vi "GSI-HVSwitch2.set operational mode.vi"(0 "i ref in":refnum<vi>, 2 "mode":T1, 3 "ms timeout (10000)":i32=10000, 5 "error in (no error)":errorcluster) -> (14 "i ref out":refnum<vi>, 17 "timed out":bool, 19 "error out":errorcluster)   [LabVIEW 2014, in "GSI-HVSwitch2.lvlib"]
doc: "Sets the operational mode of the device."
uses:
  GSI-HVSwitch2.lvlib
  GSI-HVSwitch2.mode.ctl
  CS_Core/CSApplicationBaseClasses/DeviceBase/DeviceBase.deviceState.ctl
  CS_Core/CSApplicationBaseClasses/PSChannelBase/PSChannelBase.statusType.ctl
  CSlibraries/UtilityLib/UtilityLib.valueStatus.ctl
  CS_Core/CSSystem/CoreDefs/CoreDefs.error_type.ctl
  CS_Core/CSSystem/CoreDefs/CoreDefs.error_severity.ctl
  CS_Core/CSApplicationBaseClasses/DeviceBase/DeviceBase.lvlib
  CS_Core/CSApplicationBaseClasses/PSChannelBase/PSChannelBase.lvlib
  CSlibraries/UtilityLib/UtilityLib.lvlib
  CS_Core/CSSystem/CSSystemLib/CSSystemLib.lvlib
  CS_Core/CSSystem/CoreLib/CoreLib.lvlib
  CSlibraries-extern/DimLVEvent/LVDimInterface/LVDimInterface.lvlib
  instr.lib/hvSwitch2/HVSwitch2Driver.lvlib
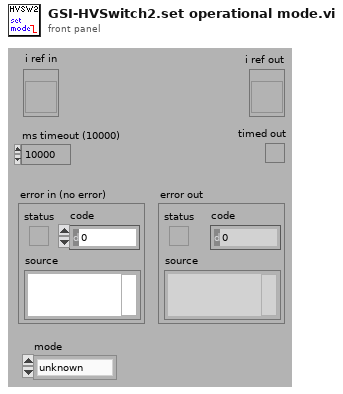
[diagram p1: front panel]
types:
  T1 = typedef "GSI-HVSwitch2.lvlib/GSI-HVSwitch2.mode.ctl" = enum16{"unknown", "switch", "stepper"}
  T2 = typedef "UtilityLib.lvlib/UtilityLib.valueStatus.ctl" = enum16{"no info available", "stand by/off", "on", "warning", "alarm/malfunction", "not implemented", "user action required", "important information", "system default", "control default", "indicator default", "button default"}
  T3 = typedef "CoreDefs.error_severity.ctl" = enum16{"undefined", "information", "warning", "error", "fatal"}
  T4 = typedef "CoreDefs.error_type.ctl" = enum16{"no error", "can't load process", "can't unload process", "process does not exist", "can't install process", "can't remove process", "unknown function", "time out", "can't execute function", "duplicate queue name", "super not found", "caller queue invalid", "can't ping process", "unknown error", "VISA Error", "VISA timeout", "GPIB timeout", "GPIB error", "communication error", "data type mismatch", "can't read data from OPC server", "can't write data to OPC server", "OET error", "function not implemented", "process already exists", "invalid Shared Variable name", "error writing Shared Variable", "error reading Shared Variable", "invalid client name", "corrupt database", "unknown class", "call not authorized", "parameter out of range", "OET timeout: can't get data to modify", "invalid queue name", "requested operation incompatible with current state", "event undefined", "event disabled", "state undefined", "caller is not a friend", "EventBuilder: bad eventID", "EventBuilder: no DAQ devices", "a thread must not stop itself", "UNUSED ELEMENT4", "DiscArchiver: eventData incomplete", "DiscArchiver: eventData does not belong to run", "DiscArchiver: can't open file", "DiscArchiver: can't write to file", "DiscArchiver: available disc space low", "can't acquire semaphore", "error reading data from database", "notifier object is not existing", "can't register process", "can't unregister process", "illegal event type", "object disabled", "object already exists", "can't change state", "Instrument not found", "no connection to remote node", "invalid reference", "N/A", "UNUSED ELEMENT 1", "element not found", "illegal TCP/IP connection detected", "object does not exist", "invalid access ID", "unknown CS system", "invalid privilige", "unsupported data type", "unsupported server type", "IO server already exists", "Shared Variable already exists"}
  T5 = typedef "GSI-HVSwitch2.lvlib/GSI-HVSwitch2.i attribute.ctl" = cluster{"SDEX VISA Cluster":T6, "SetVoltage SW0":dbl, "SetVoltage SW1":dbl, "ActTempAmp":dbl, "ActTempPS1":dbl, "ActTempPS2":dbl, "mode":T1, "interfaceInitialized":bool, "serviceIDs":cluster{"nomVoltage0ID":i32, "nomVoltage1ID":i32, "actTempAmpID":i32, "actTempPS1ID":i32, "actTempPS2ID":i32, "modeID":i32}, "usedChannels":i32}
  T6 = typedef "SDEXDriver.lvlib/SDEX.VISA Control.ctl" = cluster{"VISA resource name":refnum<visa-resource-name>, "HEX address":u16, "VISA Timeout Value (1000 ms)":u32, "Lock Timeout (1000 ms)":u32, "semaphore":T7, "Baud rate":u32, "revision":T8, "deviceInfo":string}
  T7 = typedef "Semaphore RefNum" = refnum<k1>
  T8 = typedef "SDEXDriver.lvlib/SDEX.revisionType.ctl" = enum16{"unknown", "hvamp3", "hvswi1", "htrp0", "WDG0"}
  T9 = typedef "DeviceBase.lvlib/DeviceBase.deviceState.ctl" = i16
  T10 = typedef "PSChannelBase.lvlib/PSChannelBase.statusType.ctl" = i32
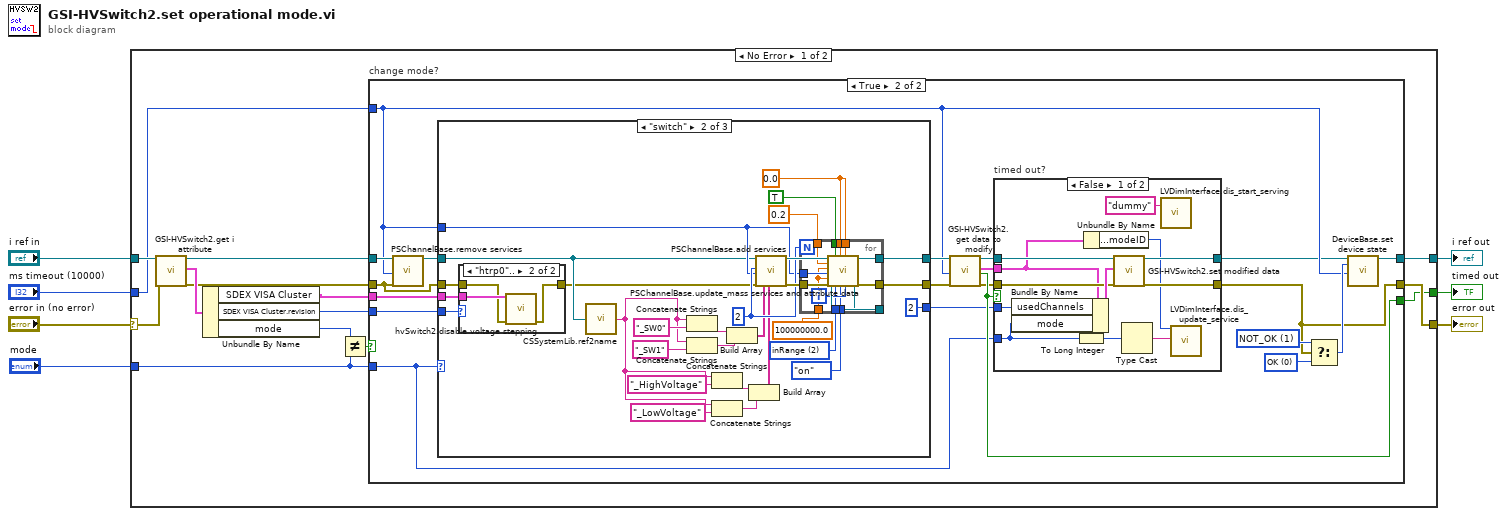
[diagram p0: block diagram]
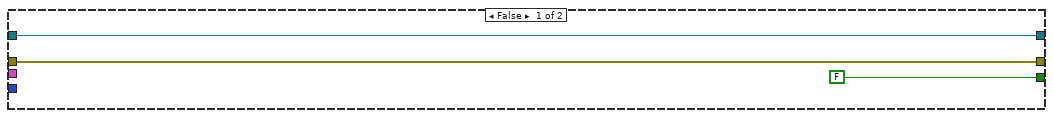
[diagram p2: hidden frame]
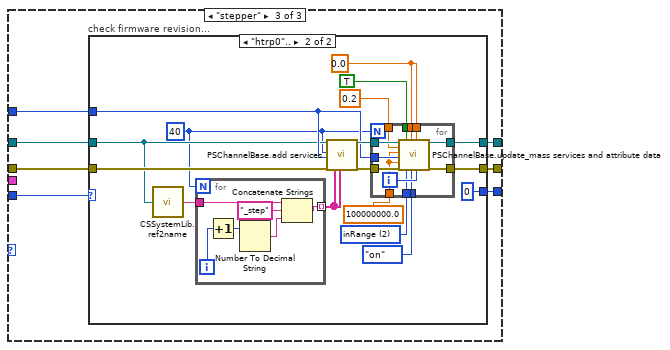
[diagram p6: hidden frame]
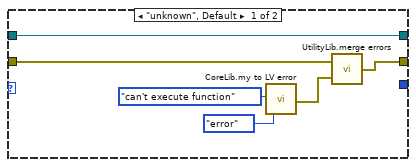
[diagram p7: hidden frame]
diagram:
  n1 = case shown="No Error" "error in (no error)" {
    selector: "error in (no error)" -> [w19 w156]
    tunnel: "i ref in" -> [w20 w157]
    tunnel: "ms timeout (10000)" -> [w11 _]
    tunnel: [w12 _] -> w5
    tunnel: [w21 w157] -> w4
    tunnel: [w13 w156] -> w3
    tunnel: "mode" -> [w10 _]
    frame No Error {
      n2 = call "GSI-HVSwitch2.get i attribute.vi"("i ref in"=w20, "error in (no error)"=w19) -> ("i ref out"=w15:refnum<vi>, "i attribute"=w18:T5, "error out"=w14:errorcluster)  [unwired: 15 in]
      n3 = Unbundle By Name(w18) -> ("SDEX VISA Cluster"=w8:T6, "SDEX VISA Cluster.revision"=w9:T8, "mode"=w17:T1)
      n4 = Not Equal?(x=w17, y=w10) -> (x != y?=w16:bool)
      n5 = case "change mode?" shown="True" w16 {
        tunnel: [w24 w44] -> w21
        tunnel: w15 -> [w24 w40]
        tunnel: w14 -> [w23 w38]
        tunnel: [w23 w29] -> w13
        tunnel: [FALSE w33] -> w12
        tunnel: w11 -> [_ w34]
        tunnel: w10 -> [_ w27]
        tunnel: w9 -> [_ w37]
        tunnel: w8 -> [_ w25]
        frame False {
        }
        frame True {
          w42 = T9 1 items=["ERROR"=-1, "OK"=0, "NOT_OK"=1] ("deviceState")
          w43 = T9 0 items=["ERROR"=-1, "OK"=0, "NOT_OK"=1] ("deviceState")
          n6 = call "PSChannelBase.remove services.vi"("i ref in"=w40, "ms timeout (10000)"=w34, "error in (no error)"=w38) -> ("i ref out"=w39:refnum<vi>)  [unwired: 14 in, 2 out]
          n7 = case shown="\"switch\"" w27 {
            tunnel: w39 -> [w60 w70 w111]
            tunnel: [w60 w68 w110] -> w36
            tunnel: w38 -> [w59 w63 w113]
            tunnel: [w59 w67 w109] -> w35
            tunnel: w34 -> [_ w71 w112]
            tunnel: w37 -> [_ w61 w108]
            tunnel: [_ 2 w107] -> w26
            tunnel: w25 -> [_ w64 _]
            frame "unknown", Default {
            }
            frame "switch" {
              w66 = 0.0
              w89 = T10 2 items=["onOff"=1, "inRange"=2, "rampingUp"=4, "rampingDown"=8, "tripped"=16, "error"=32] ("status")
              w82 = 2 ("nofChannels")
              n8 = case shown="\"htrp0\".." w61 {
                tunnel: w64 -> [_ w93]
                tunnel: w63 -> [w90 w92]
                tunnel: [w90 w91] -> w62
                frame "unknown", Default {
                }
                frame "htrp0".. {
                  n9 = call "hvSwitch2.disable voltage stepping.vi"("SDEX VISA Cluster"=w93, "error in (no error)"=w92) -> ("error out"=w91:errorcluster)  [unwired: 12 in, 1 out]
                }
              }
              n10 = call "CSSystemLib.ref2name.vi"("obj refnum"=w70) -> ("name"=w69:string)
              n11 = Concatenate Strings(w69, "_SW0" ("string")) -> (w74:string)
              n12 = Concatenate Strings(w69, "_SW1" ("string")) -> (w76:string)
              n13 = Concatenate Strings(w69, "_HighVoltage" ("string")) -> (w79:string)
              n14 = Concatenate Strings(w69, "_LowVoltage" ("string")) -> (w80:string)
              n15 = Build Array(w74, w76) -> (w75:string[])
              n16 = Build Array(w79, w80) -> (w81:string[])
              n17 = call "PSChannelBase.add services.vi"("i ref in"=w70, "nofChannels"=w82, "ms timeout (10000)"=w71, "error in (no error)"=w62, "physicalNames"=w75, "logicalNames"=w81) -> ("i ref out"=w84:refnum<vi>, "error out"=w85:errorcluster)  [unwired: 11 in, 1 out]
              n18 = for {
                N: w82 -> [_]
                tunnel: w84 -> [w106]
                tunnel: w85 -> [w105]
                tunnel: [w104] -> w68
                tunnel: [w103] -> w67
                tunnel: TRUE ("onOff") -> [w102]
                tunnel: w66 -> [w101]
                tunnel: w66 -> [w100]
                tunnel: 0.2 -> [w99]
                tunnel: w71 -> [w98]
                tunnel: 100000000.0 -> [w97]
                tunnel: UtilityLib.valueStatus."on" ("valueStatus") -> [w95]
                tunnel: w89 -> [w94]
                i -> [w96]
                n19 = call "PSChannelBase.update_mass services and attribute data.vi"("i ref in"=w106, "tripCurrent"=w99, "rampUpSpeed"=w97, "ms timeout (10000)"=w98, "rampDownSpeed"=w97, "error in (no error)"=w105, "onOff"=w102, "status"=w94, "voltage"=w101, "valueStatus"=w95, "current"=w100, "channelNumber"=w96) -> ("i ref out"=w104:refnum<vi>, "error out"=w103:errorcluster)  [unwired: 5 in, 1 out]
              }
            }
            frame "stepper" {
              n20 = case "check firmware revision..." shown="\"htrp0\".." w108 {
                tunnel: w113 -> [w119 w129]
                tunnel: w112 -> [_ w128]
                tunnel: w111 -> [w118 w127]
                tunnel: [w118 w126] -> w110
                tunnel: [w117 w125] -> w109
                tunnel: [_ 0] -> w107
                frame "unknown", Default {
                  n21 = call "CoreLib.my to LV error.vi"("ErrorTypes"=CoreDefs.error_type."can't execute function", "severityLevel"=CoreDefs.error_severity."error") -> ("myErrorCluster"=w116:errorcluster)  [unwired: 16 in, 1 out]
                  n22 = call "UtilityLib.merge errors.vi"("error2 (no error)"=w116, "error1 (no error)"=w119) -> ("error out"=w117:errorcluster)
                }
                frame "htrp0".. {
                  w124 = 0.0
                  w136 = T10 2 items=["onOff"=1, "inRange"=2, "rampingUp"=4, "rampingDown"=8, "tripped"=16, "error"=32] ("status")
                  w123 = 40 ("nofChannels")
                  n23 = call "CSSystemLib.ref2name.vi"("obj refnum"=w127) -> ("name"=w122:string)
                  n24 = for {
                    N: w123 -> [_]
                    tunnel: w122 -> [w140]
                    tunnel: [w139] -> w121 mode=indexing
                    i -> [w142]
                    n25 = Increment(x=w142) -> (x+1=w141:i32)
                    n26 = Number To Decimal String(number=w141) -> (decimal integer string=w138:string)  [unwired: 1 in]
                    n27 = Concatenate Strings(w140, "_step" ("string"), w138) -> (w139:string)
                  }
                  n28 = call "PSChannelBase.add services.vi"("i ref in"=w127, "nofChannels"=w123, "ms timeout (10000)"=w128, "error in (no error)"=w129, "physicalNames"=w121, "logicalNames"=w121) -> ("i ref out"=w131:refnum<vi>, "error out"=w132:errorcluster)  [unwired: 11 in, 1 out]
                  n29 = for {
                    N: w123 -> [_]
                    tunnel: w131 -> [w155]
                    tunnel: w132 -> [w154]
                    tunnel: [w153] -> w126
                    tunnel: [w152] -> w125
                    tunnel: TRUE ("onOff") -> [w151]
                    tunnel: w124 -> [w150]
                    tunnel: w124 -> [w149]
                    tunnel: 0.2 -> [w148]
                    tunnel: w128 -> [w147]
                    tunnel: 100000000.0 -> [w146]
                    tunnel: UtilityLib.valueStatus."on" ("valueStatus") -> [w144]
                    tunnel: w136 -> [w143]
                    i -> [w145]
                    n30 = call "PSChannelBase.update_mass services and attribute data.vi"("i ref in"=w155, "tripCurrent"=w148, "rampUpSpeed"=w146, "ms timeout (10000)"=w147, "rampDownSpeed"=w146, "error in (no error)"=w154, "onOff"=w151, "status"=w143, "voltage"=w150, "valueStatus"=w144, "current"=w149, "channelNumber"=w145) -> ("i ref out"=w153:refnum<vi>, "error out"=w152:errorcluster)  [unwired: 5 in, 1 out]
                  }
                }
              }
            }
          }
          n31 = call "GSI-HVSwitch2.get data to modify.vi"("i ref in"=w36, "ms timeout (10000)"=w34, "error in (no error)"=w35) -> ("i ref out"=w32:refnum<vi>, "i attribute"=w28:T5, "timed out"=w33:bool, "error out"=w30:errorcluster)  [unwired: 13 in]
          n32 = case "timed out?" shown="False" w33 {
            tunnel: w32 -> [w56 w58]
            tunnel: [w55 w58] -> w31
            tunnel: [w54 w57] -> w29
            tunnel: w30 -> [w52 w57]
            tunnel: w28 -> [w51 _]
            tunnel: w27 -> [w49 _]
            tunnel: w26 -> [w45 _]
            frame False {
              n33 = Bundle By Name(cluster=w51, "usedChannels"=w45, "mode"=w49) -> (w53:T5)
              n34 = To Long Integer(number=w49) -> (32bit integer=w48:i32)
              n35 = Unbundle By Name(w51) -> ("serviceIDs.modeID"=w50:i32)
              n36 = call "GSI-HVSwitch2.set modified data.vi"("i ref in"=w56, "i attribute"=w53, "error in (no error)"=w52) -> ("i ref out"=w55:refnum<vi>, "error out"=w54:errorcluster)  [unwired: 15 in]
              n37 = Type Cast(x=w48) -> (*(type *) &x=w47:string)  [unwired: 1 in]
              n38 = call "LVDimInterface.dis_start_serving.vi"("serverName"="dummy") -> ()  [unwired: 17 in, 2 out]
              n39 = call "LVDimInterface.dis_update_service.vi"("my_serviceID"=w50, "data"=w47) -> ()  [unwired: 15 in, 3 out]
            }
            frame True {
            }
          }
          n40 = Select(t=w42, s=w29, f=w43) -> (s? t:f=w41:T9)
          n41 = call "DeviceBase.set device state.vi"("i ref in"=w31, "deviceState"=w41, "ms timeout (10000)"=w34) -> ("i ref out"=w44:refnum<vi>)  [unwired: 14 in, 2 out]
        }
      }
    }
    frame Error {
    }
  }
  "error out" <- w3
  "i ref out" <- w4
  "timed out" <- w5
